vi "Updater.vi"() -> ()   [LabVIEW 2011]
uses:
  Summitek EXT/Miscellaneous/OGAB Version.ctl
  server/database/History/History Record.ctl
  server/database/Fields/Field Record.ctl
  server/database/Fields/Field DataTypes.ctl
  server/database/Fields/Field NextItem.ctl
  server/database/Stations/Instruments/Instrument Record Fields.ctl
  Summitek EXT/OpenG EXT/file/file.llb/File Exists - Scalar__ogtk.vi
  ITK EXT/http/config.llb/HTTP SRM.vi
panel:
  in  "spartan install path":path=path "C:/Development/Spartan"
  out "Database Operation":string
  out "Status":string
  out "Spartan Install Path":path
  out "ver":string
  in  "Version":T1 {"Build Date/Time" format="%<%X\n%x>T"}
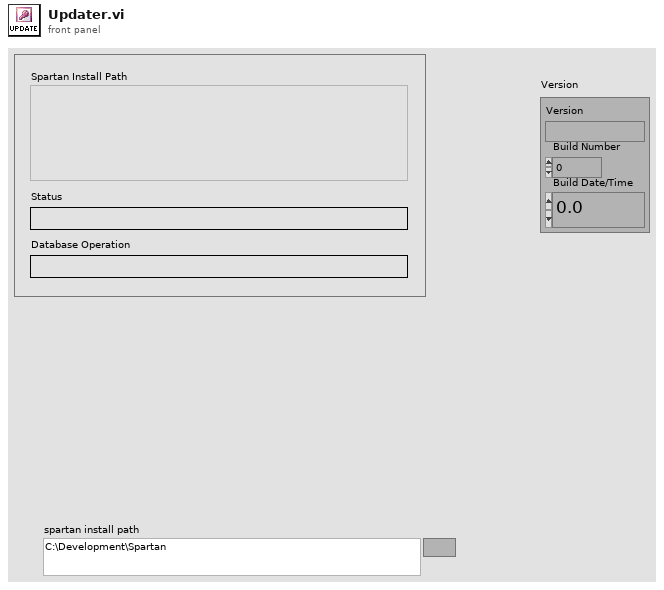
[diagram p1: front panel]
types:
  T1 = typedef "OGAB Version.ctl" = cluster{"Version":string, "Build Number":u32, "Build Date/Time":dbl}
  T2 = typedef "History Record.ctl" = cluster{"ixHistory":i32, "sVersion":string, "tUpdate":timestamp}
  T3 = typedef "Connection Refnum.ctl" = cluster{"Environment Handle":i32, "Connection Handle":i32}
  T4 = typedef "Field Record.ctl" = cluster{"ixField":i32, "iSequenceOrder":i32, "sxFieldId":string, "sxSequenceId":string, "sDisplayName":string, "sValue":string, "sUnits":string, "nDataType":T5, "nNextItem":T6, "fSystem":bool, "fSystemValue":bool, "fRequired":bool, "fSetAtTest":bool, "fTestField":bool, "fDeleted":bool, "fIndexed":bool, "fFreeList":bool}
  T5 = typedef "Field DataTypes.ctl" = enum32{"text", "numeric", "list", "timestamp", "boolean"}
  T6 = typedef "Field NextItem.ctl" = enum32{"Reset", "Retain", "Auto-Increment"}
  T7 = typedef "Instrument Record Fields.ctl" = enum32{"sxInstrumentId", "sDriverId", "sDriverType", "sSerialNumber", "tLastCalibration", "tCalibrationDue", "sConfiguration", "ixInstrument"}
  T8 = cluster{"Environment Handle":i32, "Connection Handle":i32}
  T9 = typedef "Instrument Record.ctl" = cluster{"ixInstrument":i32, "sxInstrumentId":string, "sDriverId":string, "sDriverType":string, "sSerialNumber":string, "tLastCalibration":timestamp, "tCalibrationDue":timestamp, "sConfiguration":string}
  T10 = cluster{"IndexName":string, "sxFieldId":string}[]
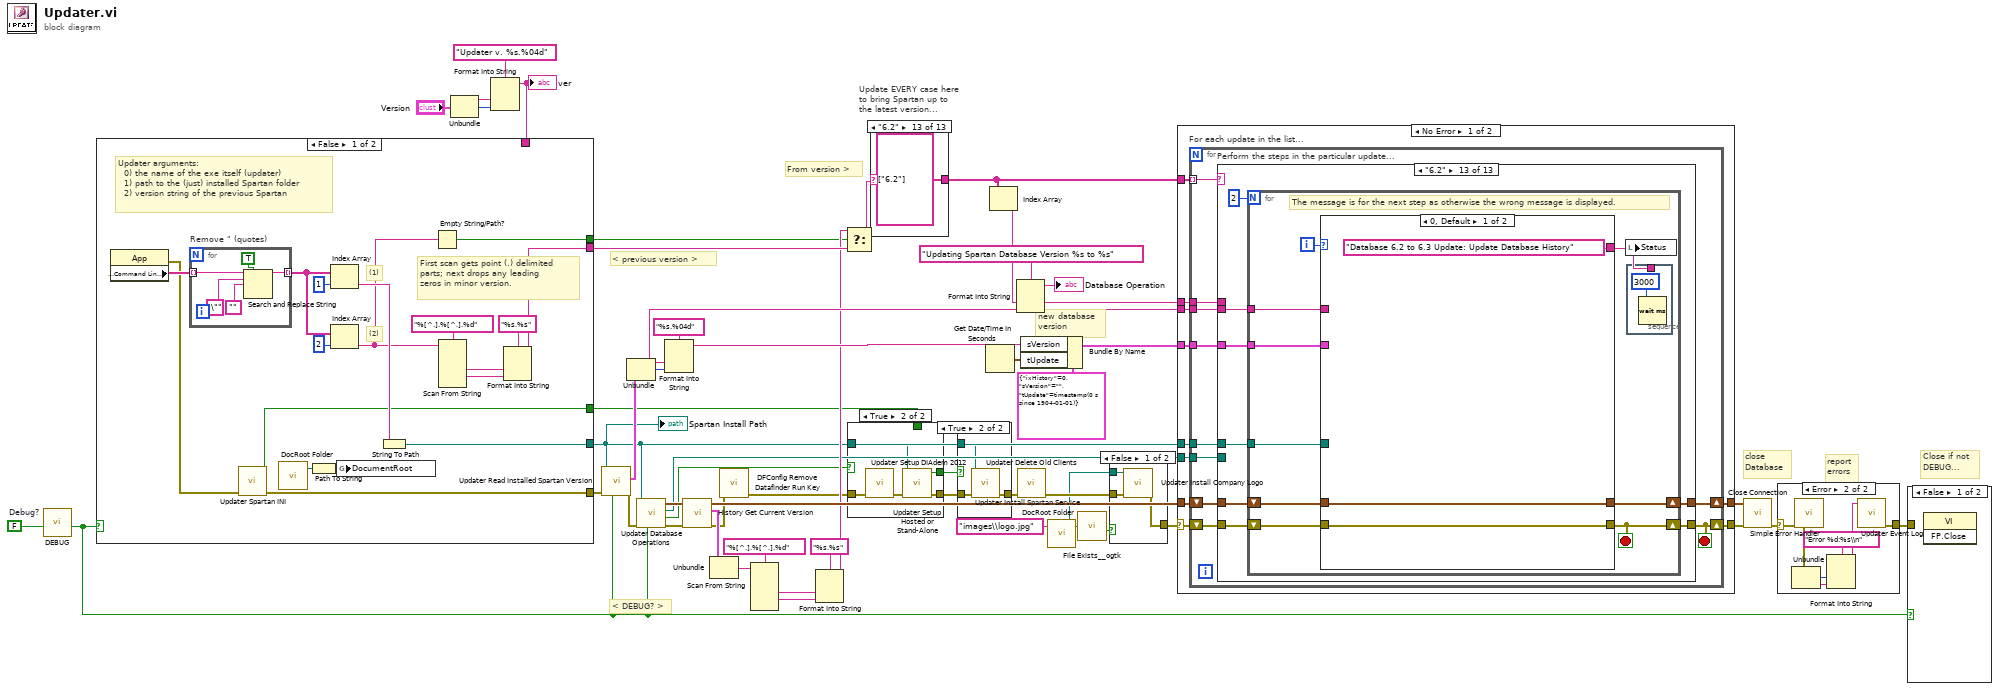
[diagram p0: block diagram]
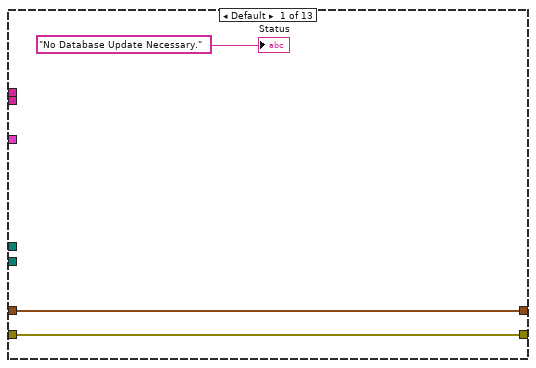
[diagram p2: hidden frame]
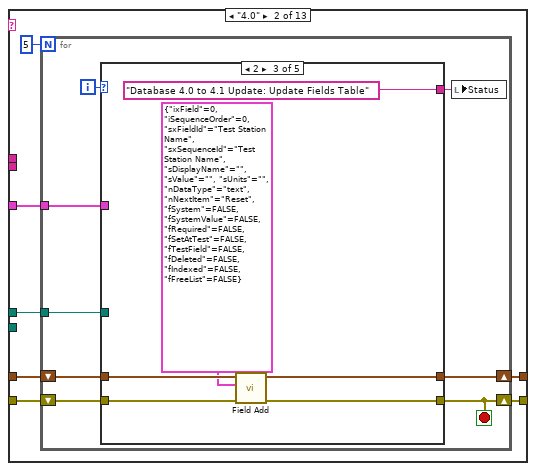
[diagram p3: hidden frame]
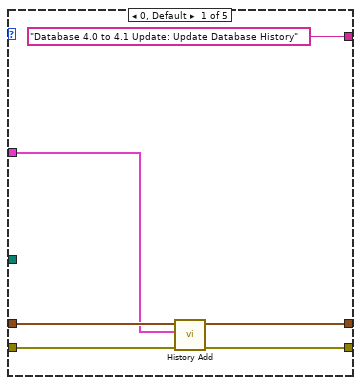
[diagram p4: hidden frame]
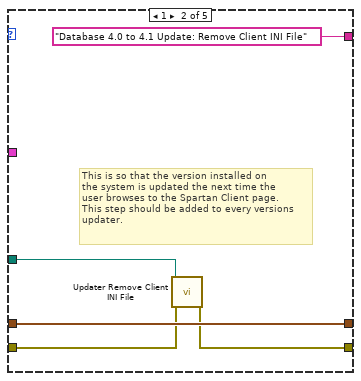
[diagram p5: hidden frame]
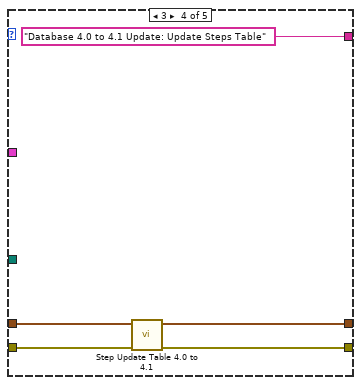
[diagram p6: hidden frame]
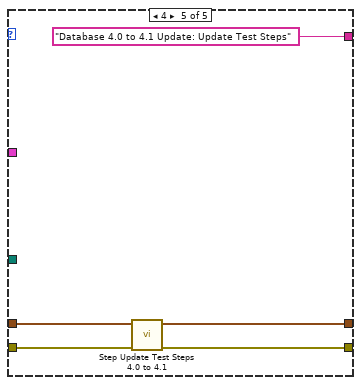
[diagram p7: hidden frame]
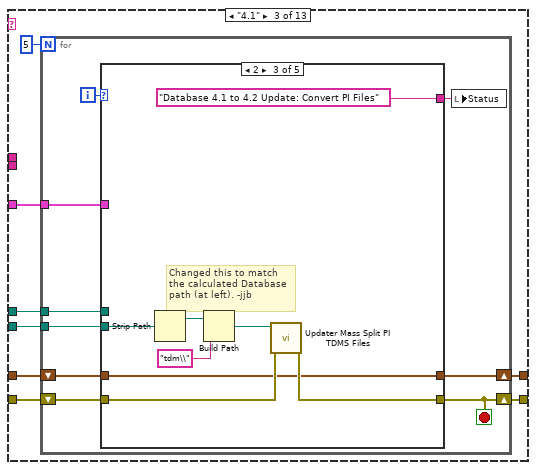
[diagram p8: hidden frame]
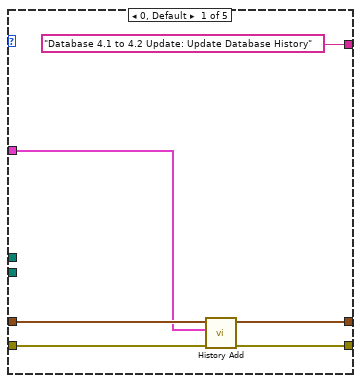
[diagram p9: hidden frame]
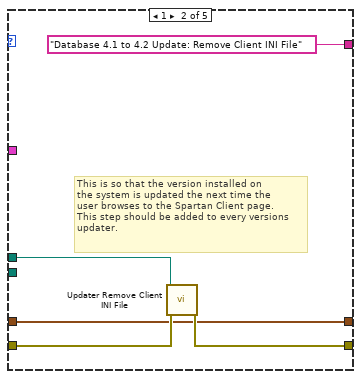
[diagram p10: hidden frame]
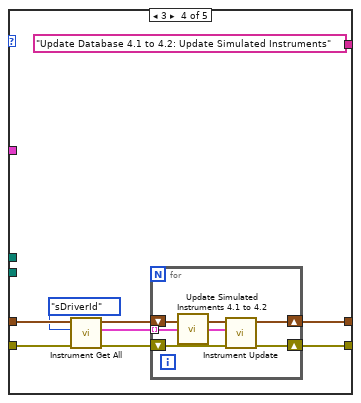
[diagram p11: hidden frame]
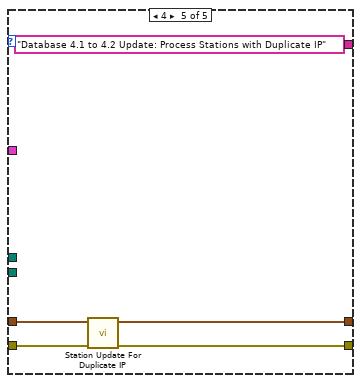
[diagram p12: hidden frame]
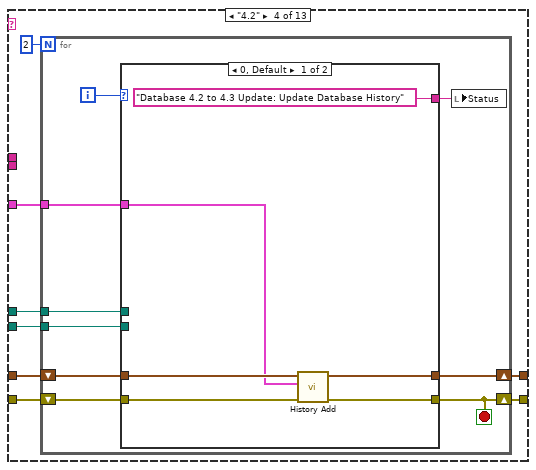
[diagram p13: hidden frame]
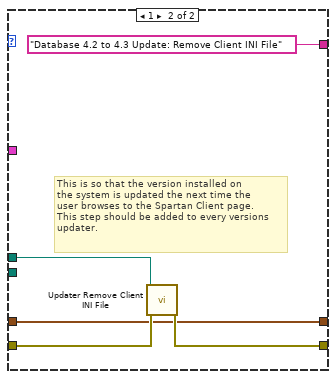
[diagram p14: hidden frame]
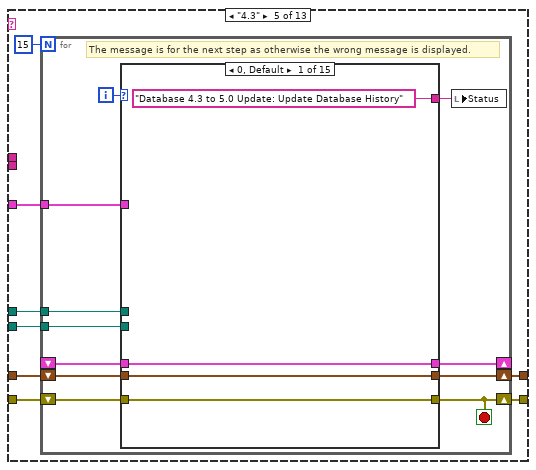
[diagram p15: hidden frame]
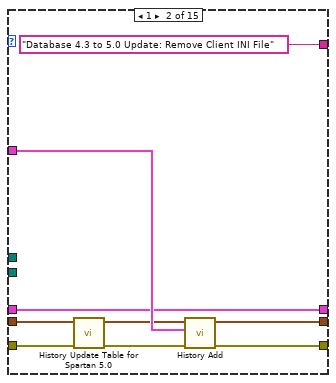
[diagram p16: hidden frame]
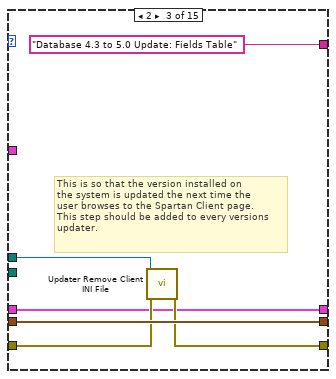
[diagram p17: hidden frame]
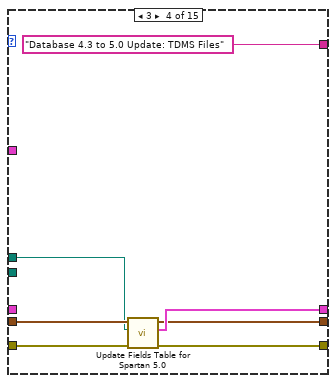
[diagram p18: hidden frame]
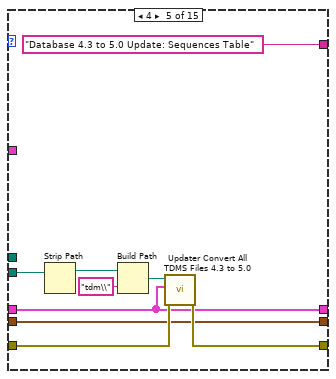
[diagram p19: hidden frame]
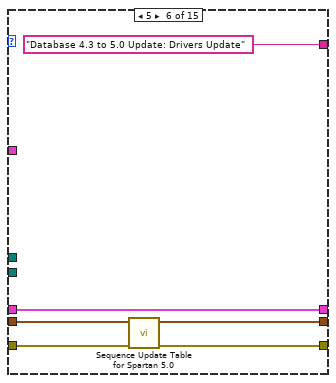
[diagram p20: hidden frame]
diagram:
  w47 = FALSE  # Debug?
  # "new database\nversion"
  # "From version >"
  # "close\nDatabase"
  # "report\nerrors"
  # "Close if not\nDEBUG..."
  # "< DEBUG? >"
  # "< previous version >"
  n1 = call "DEBUG.vi"("Dev DEBUG? (f)"=w47) -> ("DEBUG?"=w19:bool)  [unwired: 1 in, 5 out]
  n2 = Unbundle("Version") -> ("Version"=w50:string, "Build Number"=w51:u32)  [unwired: 1 out]
  n3 = Format Into String(format string="Updater v. %s.%04d", w50, w51) -> (resulting string=w45:string)  [unwired: 2 in, 1 out]
  "ver" <- w45
  n4 = case shown="False" w19 {
    tunnel: [w61 "spartan install path"] -> w9
    tunnel: [w63 "5.2"] -> w48
    tunnel: [w59 errorcluster {"status"=FALSE, "code"=0, "source"=""} ("error out")] -> w23
    tunnel: w45 -> [_ _]
    tunnel: [w56 TRUE] -> w15
    tunnel: [w55 _] -> w8
    frame False {
      # "First scan gets point (.) delimited\nparts; next drops any leading\nzeros in minor version."
      # "(2)"
      # "(1)"
      # "Updater arguments:\n  0) the name of the exe itself (updater)\n  1) path to the (just) installed Spartan folder\n  2) version string of the previous Spartan"
      n5 = property class="App"() -> (error out=w60:errorcluster, "Application:Command Line Arguments"=w70:string[])  [unwired: 2 in, 1 out]
      n6 = for "Remove \" (quotes)" {
        tunnel: w70 -> [w73] mode=indexing
        tunnel: [w72] -> w67 mode=indexing
        n7 = Search and Replace String(replace all?=TRUE, input string=w73, search string="\"", replace string="") -> (result string=w72:string)  [unwired: 1 in, 6 out]
      }
      n8 = call "Updater Spartan INI.vi"("error in (no error)"=w60) -> ("error out"=w59:errorcluster, "Run as Service?"=w55:bool)  [unwired: 9 in]
      n9 = call "DocRoot Folder.vi"() -> ("DocumentRoot Folder"=w54:path)  [unwired: 3 in]
      n10 = Path To String(path=w54) -> (string=w53:string)
      n11 = Index Array(array=w67, index=1) -> (element=w62:string)
      n12 = Index Array(array=w67, index=2) -> (element=w57:string)
      n13 = global write "HTTP SRM.vi" "DocumentRoot"(w53) -> ()
      n14 = String To Path(string=w62) -> (path=w61:path)
      n15 = Empty String/Path?(string/path=w57) -> (empty?=w56:bool)
      n16 = Scan From String(format string="%[^.].%[^.].%d", input string=w57) -> (output 1=w64:string, output 2=w58:string)  [unwired: 2 in, 7 out]
      n17 = Format Into String(format string="%s.%s", w64, w58) -> (resulting string=w63:string)  [unwired: 2 in, 1 out]
    }
    frame True {
      # "<--- DEBUGGING --->"
    }
  }
  "Spartan Install Path" <- w9
  n18 = call "Updater Read Installed Spartan Version.vi"("DEBUG? (f)"=w19, "error in (no error)"=w23, "Spartan Install Folder (empty)"=w9) -> ("error out"=w22:errorcluster, "Version"=w41:T1)  [unwired: 3 in, 4 out]
  n19 = Unbundle(w41) -> ("Version"=w33:string, "Build Number"=w43:u32)  [unwired: 1 out]
  n20 = call "Updater Database Operations.vi"("Debug (f)?"=w19, "error in (no error)"=w22, "Spartan Install Path (empty)"=w9) -> ("error out"=w21:errorcluster, "New Spartan"=w13:bool, "Spartan Database Path"=w14:path, "Connection Refnum"=w20:T3)  [unwired: 5 in]
  n21 = Format Into String(format string="%s.%04d", w33, w43) -> (resulting string=w37:string)  [unwired: 2 in, 1 out]
  n22 = call "History Get Current Version.vi"("error in (no error)"=w21, "Connection Refnum"=w20) -> ("error out"=w16:errorcluster, "Current Version Record"=w31:T2, "Connection Refnum"=w32:T3)  [unwired: 7 in]
  n23 = Unbundle(w31) -> ("sVersion"=w26:string)  [unwired: 2 out]
  n24 = call "DFConfig Remove Datafinder Run Key.vi"("error in (no error)"=w16) -> ("error out"=w7:errorcluster)  [unwired: 10 out]
  n25 = Scan From String(format string="%[^.].%[^.].%d", input string=w26) -> (output 1=w28:string, output 2=w27:string)  [unwired: 2 in, 7 out]
  n26 = Format Into String(format string="%s.%s", w28, w27) -> (resulting string=w25:string)  [unwired: 2 in, 1 out]
  n27 = Select(t=w25, s=w15, f=w48) -> (s? t:f=w24:string)
  n28 = case shown="True" w13 {
    tunnel: w7 -> [w81 w83]
    tunnel: w9 -> [_ w86]
    tunnel: [w81 w85] -> w11
    tunnel: [w80 w84] -> w12
    tunnel: w8 -> [w80 _]
    frame False {
    }
    frame True {
      n29 = call "Updater Setup DIAdem 2012.vi"("error in (no error)"=w83) -> ("error out"=w82:errorcluster)  [unwired: 10 in]
      n30 = call "Updater Setup Hosted or Stand-Alone.vi"("error in (no error)"=w82, "Spartan Install Path (empty)"=w86) -> ("error out"=w85:errorcluster, "Hosted?"=w84:bool)  [unwired: 8 in]
    }
  }
  n31 = case "Update EVERY case here\nto bring Spartan up to\nthe latest version..." shown="\"6.2\"" w24 {
    tunnel: [string[] ["New Installation"] string[] ["4.0", "4.1", "4.2", "4.3", "5.0", "5.1", "5.2", "5.3", "5.4", "6.0", "6.1", "6.2"] string[] ["4.1", "4.2", "4.3", "5.0", "5.1", "5.2", "5.3", "5.4", "6.0", "6.1", "6.2"] string[] ["4.2", "4.3", "5.0", "5.1", "5.2", "5.3", "5.4", "6.0", "6.1", "6.2"] string[] ["4.3", "5.0", "5.1", "5.2", "5.3", "5.4", "6.0", "6.1", "6.2"] string[] ["5.0", "5.1", "5.2", "5.3", "5.4", "6.0", "6.1", "6.2"] string[] ["5.1", "5.2", "5.3", "5.4", "6.0", "6.1", "6.2"] string[] ["5.2", "5.3", "5.4", "6.0", "6.1", "6.2"] string[] ["5.3", "5.4", "6.0", "6.1", "6.2"] string[] ["5.4", "6.0", "6.1", "62."] string[] ["6.0", "6.1", "6.2"] string[] ["6.1", "6.2"] string[] ["6.2"]] -> w2
    frame Default {
    }
    frame "4.0" {
    }
    frame "4.1" {
    }
    frame "4.2" {
    }
    frame "4.3" {
    }
    frame "5.0" {
    }
    frame "5.1" {
    }
    frame "5.2" {
    }
    frame "5.3" {
    }
    frame "5.4" {
    }
    frame "6.0" {
    }
    frame "6.1" {
    }
    frame "6.2" {
    }
  }
  n32 = case shown="True" w12 {
    tunnel: w11 -> [w100 w102]
    tunnel: [w100 w103] -> w10
    tunnel: w9 -> [_ w101]
    frame False {
    }
    frame True {
      n33 = call "Updater Install Spartan Service.vi"("error in (no error)"=w102, "Spartan Install Path"=w101) -> ("error out"=w103:errorcluster)  [unwired: 9 in]
    }
  }
  n34 = Get Date/Time In Seconds() -> (seconds since 1Jan1904=w40:timestamp)
  n35 = Index Array(array=w2) -> (element=w18:string)  [unwired: 1 in]
  n36 = Format Into String(format string="Updating Spartan Database Version %s to %s", w18, w33) -> (resulting string=→"Database Operation":string)  [unwired: 2 in, 1 out]
  n37 = call "Updater Delete Old Clients.vi"("error in (no error)"=w10) -> ("error out"=w6:errorcluster)  [unwired: 10 in]
  n38 = Bundle By Name(cluster=T2 {"ixHistory"=0, "sVersion"="", "tUpdate"=timestamp(0 s since 1904-01-01)} ("Auto_Number Record"), "sVersion"=w37, "tUpdate"=w40) -> (w38:T2)
  n39 = call "DocRoot Folder.vi"("Relative Path (\"\" - Folder)"="images\\logo.jpg" ("Relative Path (\"\" - Folder)")) -> ("DocumentRoot Folder"=w3:path)  [unwired: 2 in]
  n40 = call-poly "File Exists__ogtk.vi"("file path"=w3) -> ("exists"=w4:bool)  [unwired: 6 in, 1 out]
  n41 = case shown="False" w4 {
    tunnel: w6 -> [w106 w107]
    tunnel: [w105 w107] -> w1
    tunnel: w3 -> [w104 _]
    frame False {
      n42 = call "Updater Install Company Logo.vi"("error in (no error)"=w106, "Path to File"=w104) -> ("error out"=w105:errorcluster)  [unwired: 9 in]
    }
    frame True {
    }
  }
  n43 = case shown="No Error" w1 {
    selector: w1 -> [w108 w655]
    tunnel: w38 -> [w117 _]
    tunnel: [w116 w655] -> w36
    tunnel: [w115 w656] -> w35
    tunnel: w33 -> [w114 _]
    tunnel: w32 -> [w113 w656]
    tunnel: w18 -> [w112 _]
    tunnel: w14 -> [w111 _]
    tunnel: w9 -> [w110 _]
    tunnel: w2 -> [w109 _]
    frame No Error {
      n44 = for "For each update in the list..." {
        tunnel: w109 -> [w127] mode=indexing
        tunnel: w117 -> [w126]
        shift-right: [w123] -> w115
        shift-left: w113 -> [w125]
        shift-right: [w118] -> w116
        shift-left: w108 -> [w124]
        tunnel: w111 -> [w122]
        tunnel: w110 -> [w121]
        tunnel: w112 -> [w120]
        tunnel: w114 -> [w119]
        stop <- w118 stop-if-true
        n45 = case "Perform the steps in the particular update..." shown="\"6.2\"" w127 {
          tunnel: w124 -> [w129 w133 w178 w234 w262 w368 w416 w450 w490 w537 w582 w608 w634]
          tunnel: w125 -> [w128 w134 w177 w233 w261 w367 w415 w449 w489 w536 w581 w607 w633]
          tunnel: [w129 w135 w176 w232 w260 w366 w414 w448 w488 w535 w580 w606 w632] -> w118
          tunnel: w126 -> [_ w136 w179 w235 w263 w369 w417 w451 w491 w538 w583 w609 w635]
          tunnel: [w128 w132 w175 w231 w259 w365 w413 w447 w487 w534 w579 w605 w631] -> w123
          tunnel: w122 -> [_ _ w174 w230 w258 w364 _ _ _ _ _ _ _]
          tunnel: w121 -> [_ w131 w173 w229 w257 w363 _ w446 w486 w533 w578 w604 w630]
          tunnel: w120 -> [_ _ _ _ _ w362 _ _ _ _ _ _ _]
          tunnel: w119 -> [_ _ _ _ _ w361 w412 w445 w485 w532 w577 w603 w629]
          frame Default {
            "Status" <- "No Database Update Necessary." ("Status")
          }
          frame "4.0" {
            n46 = for {
              N: 5 -> [_]
              tunnel: w136 -> [w144]
              shift-right: [w138] -> w135
              shift-left: w133 -> [w141]
              shift-right: [w140] -> w132
              shift-left: w134 -> [w142]
              tunnel: w131 -> [w139]
              i -> [w145]
              stop <- w138 stop-if-true
              n47 = case shown="2" w145 {
                tunnel: w142 -> [w150 w155 w162 w165 w171]
                tunnel: w141 -> [w149 w154 w161 w166 w172]
                tunnel: [w151 w153 w160 w167 w169] -> w138
                tunnel: w144 -> [w146 _ _ _ _]
                tunnel: ["Database 4.0 to 4.1 Update: Update Database History" "Database 4.0 to 4.1 Update: Remove Client INI File" "Database 4.0 to 4.1 Update: Update Fields Table" "Database 4.0 to 4.1 Update: Update Steps Table" "Database 4.0 to 4.1 Update: Update Test Steps"] -> w143
                tunnel: [w147 w155 w157 w163 w168] -> w140
                tunnel: w139 -> [_ w152 _ _ _]
                frame 0, Default {
                  n48 = call "History Add.vi"("error in (no error)"=w149, "History Record"=w146, "Connection Refnum"=w150) -> ("error out"=w151:errorcluster, "Connection Refnum"=w147:T3)  [unwired: 7 out]
                }
                frame 1 {
                  # "This is so that the version installed on\nthe system is updated the next time the\nuser browses to the Spartan Client page.\nThis step should be added to every versions\nupdater."
                  n49 = call "Updater Remove Client INI File.vi"("error in (no error)"=w154, "Spartan Install Path"=w152) -> ("error out"=w153:errorcluster)  [unwired: 9 out]
                }
                frame 2 {
                  n50 = call "Field Add.vi"("error in (no error)"=w161, "Field Record"=T4 {"ixField"=0, "iSequenceOrder"=0, "sxFieldId"="Test Station Name", "sxSequenceId"="Test Station Name", "sDisplayName"="", "sValue"="", "sUnits"="", "nDataType"=enum."text", "nNextItem"=enum."Reset", "fSystem"=FALSE, "fSystemValue"=FALSE, "fRequired"=FALSE, "fSetAtTest"=FALSE, "fTestField"=FALSE, "fDeleted"=FALSE, "fIndexed"=FALSE, "fFreeList"=FALSE}, "Connection Refnum"=w162) -> ("error out"=w160:errorcluster, "Connection Refnum"=w157:T3)  [unwired: 1 in, 6 out]
                }
                frame 3 {
                  n51 = call "Step Update Table 4.0 to 4.1.vi"("error in (no error)"=w166, "Connection Refnum"=w165) -> ("error out"=w167:errorcluster, "Connection Refnum Out"=w163:T8)  [unwired: 8 out]
                }
                frame 4 {
                  n52 = call "Step Update Test Steps 4.0 to 4.1.vi"("error in (no error)"=w172, "Connection Refnum"=w171) -> ("error out"=w169:errorcluster, "Connection Refnum Out"=w168:T8)  [unwired: 8 out]
                }
              }
              n53 = local write "Status"(w143) -> ()
            }
          }
          frame "4.1" {
            n54 = for {
              N: 5 -> [_]
              tunnel: w179 -> [w188]
              shift-right: [w184] -> w175
              shift-left: w177 -> [w185]
              shift-right: [w181] -> w176
              shift-left: w178 -> [w186]
              tunnel: w174 -> [w183]
              tunnel: w173 -> [w182]
              i -> [w189]
              stop <- w181 stop-if-true
              n55 = case shown="2" w189 {
                tunnel: w185 -> [w194 w197 w205 w215 w227]
                tunnel: w186 -> [w193 w199 w207 w216 w228]
                tunnel: [w195 w198 w206 w212 w226] -> w181
                tunnel: w188 -> [w191 _ _ _ _]
                tunnel: ["Database 4.1 to 4.2 Update: Update Database History" "Database 4.1 to 4.2 Update: Remove Client INI File" "Database 4.1 to 4.2 Update: Convert PI Files" "Update Database 4.1 to 4.2: Update Simulated Instruments" "Database 4.1 to 4.2 Update: Process Stations with Duplicate IP"] -> w187
                tunnel: [w190 w197 w205 w210 w225] -> w184
                tunnel: w183 -> [_ _ w202 _ _]
                tunnel: w182 -> [_ w196 _ _ _]
                frame 0, Default {
                  n56 = call "History Add.vi"("error in (no error)"=w193, "History Record"=w191, "Connection Refnum"=w194) -> ("error out"=w195:errorcluster, "Connection Refnum"=w190:T3)  [unwired: 7 out]
                }
                frame 1 {
                  # "This is so that the version installed on\nthe system is updated the next time the\nuser browses to the Spartan Client page.\nThis step should be added to every versions\nupdater."
                  n57 = call "Updater Remove Client INI File.vi"("error in (no error)"=w199, "Spartan Install Path"=w196) -> ("error out"=w198:errorcluster)  [unwired: 9 out]
                }
                frame 2 {
                  # "Changed this to match\nthe calculated Database\npath (at left). -jjb"
                  n58 = Strip Path(path=w202) -> (stripped path=w203:path)  [unwired: 1 out]
                  n59 = Build Path(base path=w203, name or relative path="tdm\\") -> (appended path=w201:path)
                  n60 = call "Updater Mass Split PI TDMS Files.vi"("error in (no error)"=w207, "Spartan TDM Path"=w201) -> ("error out"=w206:errorcluster)  [unwired: 9 out]
                }
                frame 3 {
                  n61 = call "Instrument Get All.vi"("error in (no error)"=w216, "Sort by (sxInstrumentId)"=Instrument_Record_Fields."sDriverId" ("Sort by (Instrument_ID)"), "Connection Refnum"=w215) -> ("error out"=w213:errorcluster, "Instruments"=w209:T9[], "Connection Refnum"=w211:T3)  [unwired: 1 in, 5 out]
                  n62 = for {
                    shift-right: [w222] -> w212
                    shift-left: w213 -> [w223]
                    tunnel: w209 -> [w219] mode=indexing
                    shift-right: [w220] -> w210
                    shift-left: w211 -> [w221]
                    n63 = call "Update Simulated Instruments 4.1 to 4.2.vi"("Instrument Information"=w219) -> ("updated Instrument"=w218:T9)  [unwired: 2 in, 6 out]
                    n64 = call "Instrument Update.vi"("error in (no error)"=w223, "Instrument Record"=w218, "Connection Refnum"=w221) -> ("error out"=w222:errorcluster, "Connection Refnum"=w220:T3)  [unwired: 7 out]
                  }
                }
                frame 4 {
                  n65 = call "Station Update For Duplicate IP.vi"("error in (no error)"=w228, "Connection Refnum"=w227) -> ("error out"=w226:errorcluster, "Connection Refnum"=w225:T3)  [unwired: 8 out]
                }
              }
              n66 = local write "Status"(w187) -> ()
            }
          }
          frame "4.2" {
            n67 = for {
              N: 2 -> [_]
              tunnel: w235 -> [w244]
              shift-right: [w240] -> w231
              shift-left: w233 -> [w241]
              shift-right: [w237] -> w232
              shift-left: w234 -> [w242]
              tunnel: w230 -> [w239]
              tunnel: w229 -> [w238]
              i -> [w245]
              stop <- w237 stop-if-true
              n68 = case shown="0, Default" w245 {
                tunnel: w241 -> [w250 w253]
                tunnel: w242 -> [w249 w256]
                tunnel: [w251 w255] -> w237
                tunnel: w244 -> [w247 _]
                tunnel: ["Database 4.2 to 4.3 Update: Update Database History" "Database 4.2 to 4.3 Update: Remove Client INI File"] -> w243
                tunnel: [w246 w253] -> w240
                tunnel: w239 -> [_ _]
                tunnel: w238 -> [_ w252]
                frame 0, Default {
                  n69 = call "History Add.vi"("error in (no error)"=w249, "History Record"=w247, "Connection Refnum"=w250) -> ("error out"=w251:errorcluster, "Connection Refnum"=w246:T3)  [unwired: 7 out]
                }
                frame 1 {
                  # "This is so that the version installed on\nthe system is updated the next time the\nuser browses to the Spartan Client page.\nThis step should be added to every versions\nupdater."
                  n70 = call "Updater Remove Client INI File.vi"("error in (no error)"=w256, "Spartan Install Path"=w252) -> ("error out"=w255:errorcluster)  [unwired: 9 out]
                }
              }
              n71 = local write "Status"(w243) -> ()
            }
          }
          frame "4.3" {
            n72 = for {
              N: 15 -> [_]
              tunnel: w263 -> [w274]
              shift-right: [w270] -> w259
              shift-left: w261 -> [w271]
              shift-right: [w265] -> w260
              shift-left: w262 -> [w272]
              tunnel: w258 -> [w269]
              tunnel: w257 -> [w268]
              shift-right: [w267] -> _
              shift-left: _ -> [w266]
              i -> [w275]
              stop <- w265 stop-if-true
              # "The message is for the next step as otherwise the wrong message is displayed."
              n73 = case shown="0, Default" w275 {
                tunnel: w271 -> [w279 w283 w293 w297 w304 w311 w318 w323 w328 w333 w338 w343 w348 w353 w360]
                tunnel: w272 -> [w278 w282 w292 w300 w310 w315 w321 w326 w331 w336 w341 w346 w351 w356 w357]
                tunnel: [w278 w286 w291 w299 w309 w314 w320 w325 w330 w335 w340 w345 w350 w355 w358] -> w265
                tunnel: w274 -> [_ w288 _ _ _ _ _ _ _ _ _ _ _ _ _]
                tunnel: ["Database 4.3 to 5.0 Update: Update Database History" "Database 4.3 to 5.0 Update: Remove Client INI File" "Database 4.3 to 5.0 Update: Fields Table" "Database 4.3 to 5.0 Update: TDMS Files" "Database 4.3 to 5.0 Update: Sequences Table" "Database 4.3 to 5.0 Update: Drivers Update" "Database 4.3 to 5.0 Update: Tests Table" "Database 4.3 to 5.0 Update: Associations Table" "Database 4.3 to 5.0 Update: Instruments Table" "Database 4.3 to 5.0 Update: Stations Table" "Database 4.3 to 5.0 Update: Auto Number Table" "Database 4.3 to 5.0 Update: Users Table" "Database 4.3 to 5.0 Update: Steps Table" "Database 4.3 to 5.0 Update: Templates Table" _] -> w273
                tunnel: [w279 w287 w293 w296 w304 w312 w319 w324 w329 w334 w339 w344 w349 w354 w359] -> w270
                tunnel: w269 -> [_ _ _ _ w306 _ _ _ _ _ _ _ _ _ _]
                tunnel: w268 -> [_ _ w290 w295 _ _ _ _ _ _ _ _ _ _ _]
                tunnel: [w276 w284 w289 w298 w303 w313 _ _ _ _ _ _ _ _ _] -> w267
                tunnel: w266 -> [w276 w284 w289 _ w303 w313 _ _ _ _ _ _ _ _ _]
                frame 0, Default {
                }
                frame 1 {
                  n74 = call "History Update Table for Spartan 5.0.vi"("error in (no error)"=w282, "Connection Refnum"=w283) -> ("error out"=w280:errorcluster, "Connection Refnum"=w281:T3)  [unwired: 8 out]
                  n75 = call "History Add.vi"("error in (no error)"=w280, "History Record"=w288, "Connection Refnum"=w281) -> ("error out"=w286:errorcluster, "Connection Refnum"=w287:T3)  [unwired: 7 out]
                }
                frame 2 {
                  # "This is so that the version installed on\nthe system is updated the next time the\nuser browses to the Spartan Client page.\nThis step should be added to every versions\nupdater."
                  n76 = call "Updater Remove Client INI File.vi"("error in (no error)"=w292, "Spartan Install Path"=w290) -> ("error out"=w291:errorcluster)  [unwired: 9 out]
                }
                frame 3 {
                  n77 = call "Update Fields Table for Spartan 5.0.vi"("error in (no error)"=w300, "spartan install dir"=w295, "Connection Refnum"=w297) -> ("error out"=w299:errorcluster, "Map IndexName to FieldId"=w298:T10, "dup Connection Refnum"=w296:T3)  [unwired: 6 out]
                }
                frame 4 {
                  n78 = Strip Path(path=w306) -> (stripped path=w307:path)  [unwired: 1 out]
                  n79 = Build Path(base path=w307, name or relative path="tdm\\") -> (appended path=w305:path)
                  n80 = call "Updater Convert All TDMS Files 4.3 to 5.0.vi"("error in (no error)"=w310, "Map IndexName to FieldId"=w303, "Folder Path"=w305) -> ("error out"=w309:errorcluster)  [unwired: 8 out]
                }
                frame 5 {
                  n81 = call "Sequence Update Table for Spartan 5.0.vi"("error in (no error)"=w315, "Connection Refnum"=w311) -> ("error out"=w314:errorcluster, "Connection Refnum"=w312:T3)  [unwired: 8 out]
                }
                frame 6 {
                  n82 = call "Driver Update Table for Spartan 5.0.vi"("error in (no error)"=w321, "Connection Refnum"=w318) -> ("error out"=w320:errorcluster, "dup Connection Refnum"=w319:T3)  [unwired: 8 out]
                }
                frame 7 {
                  n83 = call "Test Update Table for Spartan 5.0.vi"("error in (no error)"=w326, "Connection Refnum"=w323) -> ("error out"=w325:errorcluster, "Connection Refnum"=w324:T3)  [unwired: 8 out]
                }
                frame 8 {
                  n84 = call "Association Update Table for Spartan 5.0.vi"("error in (no error)"=w331, "Connection Refnum"=w328) -> ("error out"=w330:errorcluster, "Connection Refnum"=w329:T3)  [unwired: 8 out]
                }
                frame 9 {
                  n85 = call "Instrument Update Table for Spartan 5.0.vi"("error in (no error)"=w336, "Connection Refnum"=w333) -> ("error out"=w335:errorcluster, "Connection Refnum"=w334:T3)  [unwired: 8 out]
                }
                frame 10 {
                  n86 = call "Station Update Table for Spartan 5.0.vi"("error in (no error)"=w341, "Connection Refnum"=w338) -> ("error out"=w340:errorcluster, "Connection Refnum"=w339:T3)  [unwired: 8 out]
                }
                frame 11 {
                  n87 = call "Auto Number Update Table for Spartan 5.0.vi"("error in (no error)"=w346, "Connection Refnum"=w343) -> ("error out"=w345:errorcluster, "Connection Refnum"=w344:T3)  [unwired: 8 out]
                }
                frame 12 {
                  n88 = call "User Update Table for Spartan 5.0.vi"("error in (no error)"=w351, "Connection Refnum"=w348) -> ("error out"=w350:errorcluster, "Connection Refnum"=w349:T3)  [unwired: 8 out]
                }
                frame 13 {
                  n89 = call "Step Update Table 4.3 to 5.0.vi"("error in (no error)"=w356, "Connection Refnum"=w353) -> ("error out"=w355:errorcluster, "Connection Refnum"=w354:T3)  [unwired: 8 out]
                }
                frame 14 {
                  n90 = call "Update Templates Table for Spartan 5.0.vi"("error in (no error)"=w357, "Connection Refnum"=w360) -> ("error out"=w358:errorcluster, "Connection Refnum"=w359:T3)  [unwired: 8 out]
                }
              }
              n91 = local write "Status"(w273) -> ()
            }
          }
          frame "5.0" {
            n92 = for {
              N: 5 -> [_]
              tunnel: w369 -> [w380]
              shift-right: [w376] -> w365
              shift-left: w367 -> [w377]
              shift-right: [w371] -> w366
              shift-left: w368 -> [w378]
              tunnel: w364 -> [w375]
              tunnel: w363 -> [w374]
              tunnel: w362 -> [w373]
              tunnel: w361 -> [w372]
              i -> [w381]
              stop <- w371 stop-if-true
              # "The message is for the next step as otherwise the wrong message is displayed."
              n93 = case shown="2" w381 {
                tunnel: w377 -> [w384 w386 w392 w405 w409]
                tunnel: w378 -> [w383 w385 w401 w407 w411]
                tunnel: [w383 w388 w400 w406 w410] -> w371
                tunnel: w380 -> [_ w390 _ _ _]
                tunnel: ["Database 5.0 to 5.1 Update: Update Database History" "Database 5.0 to 5.1 Update: TDMS Files" "Database 5.0 to 5.1 Update: Fields" "Database 5.0 to 5.1 Update: Steps" _] -> w379
                tunnel: [w384 w389 w391 w404 w408] -> w376
                tunnel: w375 -> [_ _ w397 _ _]
                tunnel: w374 -> [_ _ _ w403 _]
                tunnel: w373 -> [_ _ w394 _ _]
                tunnel: w372 -> [_ _ w393 _ _]
                frame 0, Default {
                }
                frame 1 {
                  n94 = call "History Add.vi"("error in (no error)"=w385, "History Record"=w390, "Connection Refnum"=w386) -> ("error out"=w388:errorcluster, "Connection Refnum"=w389:T3)  [unwired: 7 out]
                }
                frame 2 {
                  n95 = Strip Path(path=w397) -> (stripped path=w398:path)  [unwired: 1 out]
                  n96 = Build Path(base path=w398, name or relative path="tdm\\") -> (appended path=w396:path)
                  n97 = call "Updater Convert All TDMS Files 5.0 to 5.1.vi"("Current Version"=w393, "Connection Refnum In"=w392, "Previous Version"=w394, "error in (no error)"=w401, "Folder Path"=w396) -> ("error out"=w400:errorcluster, "Connection Refnum Out"=w391:T3)  [unwired: 5 out]
                }
                frame 3 {
                  n98 = call "Update Fields Table for Spartan 5.1.vi"("error in (no error)"=w407, "Spartan Install Dir"=w403, "Connection Refnum"=w405) -> ("error out"=w406:errorcluster, "Connection Refnum"=w404:T3)  [unwired: 7 out]
                }
                frame 4 {
                  n99 = call "Step Update Table 5.0 to 5.1.vi"("error in (no error)"=w411, "Connection Refnum"=w409) -> ("error out"=w410:errorcluster, "Connection Refnum"=w408:T3)  [unwired: 1 in, 7 out]
                }
              }
              n100 = local write "Status"(w379) -> ()
            }
          }
          frame "5.1" {
            n101 = for {
              N: 4 -> [_]
              tunnel: w417 -> [w425]
              shift-right: [w421] -> w413
              shift-left: w415 -> [w422]
              shift-right: [w419] -> w414
              shift-left: w416 -> [w423]
              tunnel: w412 -> [w420]
              i -> [w426]
              stop <- w419 stop-if-true
              # "The message is for the next step as otherwise the wrong message is displayed."
              n102 = case shown="0, Default" w426 {
                tunnel: w422 -> [w429 w431 w438 w442]
                tunnel: w423 -> [w428 w430 w440 w444]
                tunnel: [w428 w433 w439 w443] -> w419
                tunnel: w425 -> [_ w435 _ _]
                tunnel: ["Database 5.1 to 5.2 Update: Update Database History" "Database 5.1 to 5.2 Update: Fields" "Database 5.1 to 5.2 Update: Step Associations" _] -> w424
                tunnel: [w429 w434 w437 w441] -> w421
                tunnel: w420 -> [_ _ _ _]
                frame 0, Default {
                }
                frame 1 {
                  n103 = call "History Add.vi"("error in (no error)"=w430, "History Record"=w435, "Connection Refnum"=w431) -> ("error out"=w433:errorcluster, "Connection Refnum"=w434:T3)  [unwired: 7 out]
                }
                frame 2 {
                  n104 = call "Update Fields Table for Spartan 5.2.vi"("error in (no error)"=w440, "Connection Refnum"=w438) -> ("error out"=w439:errorcluster, "Connection Refnum"=w437:T3)  [unwired: 8 in]
                }
                frame 3 {
                  n105 = call "Update Add Step Associations Table for Spartan 5.2.vi"("error in (no error)"=w444, "Connection Refnum"=w442) -> ("error out"=w443:errorcluster, "Connection Refnum"=w441:T3)  [unwired: 8 in]
                }
              }
              n106 = local write "Status"(w424) -> ()
            }
          }
          frame "5.2" {
            n107 = for {
              N: 5 -> [_]
              tunnel: w451 -> [w460]
              shift-right: [w457] -> w447
              shift-left: w449 -> [w458]
              shift-right: [w453] -> w448
              shift-left: w450 -> [w459]
              tunnel: w446 -> [w456]
              tunnel: w445 -> [w455]
              i -> [w461]
              stop <- w453 stop-if-true
              # "The message is for the next step as otherwise the wrong message is displayed."
              n108 = case shown="0, Default" w461 {
                tunnel: w458 -> [w465 w467 w476 w479 w482]
                tunnel: w459 -> [w464 w466 w475 w481 w484]
                tunnel: [w464 w469 w473 w480 w483] -> w453
                tunnel: w460 -> [_ w471 _ _ _]
                tunnel: ["Database 5.2 to 5.3 Update: Update Database History" "Uninstall CrypKey Software" "Update S Parameter Fields Units" "Setup DIAdem 2010" _] -> w454
                tunnel: [w465 w470 w476 w478 w482] -> w457
                tunnel: w456 -> [_ _ w474 _ _]
                tunnel: w455 -> [_ _ _ _ _]
                frame 0, Default {
                }
                frame 1 {
                  n109 = call "History Add.vi"("error in (no error)"=w466, "History Record"=w471, "Connection Refnum"=w467) -> ("error out"=w469:errorcluster, "Connection Refnum"=w470:T3)  [unwired: 7 out]
                }
                frame 2 {
                  n110 = call "Updater Uninstall CrypKey.vi"("error in (no error)"=w475, "Spartan Install Path"=w474) -> ("error out"=w473:errorcluster)  [unwired: 9 in]
                }
                frame 3 {
                  n111 = call "Update Fields Table for Spartan 5.3.vi"("error in (no error)"=w481, "Connection Refnum"=w479) -> ("error out"=w480:errorcluster, "Connection Refnum"=w478:T3)  [unwired: 8 in]
                }
                frame 4 {
                  n112 = call "Updater Setup DIAdem 2012.vi"("error in (no error)"=w484) -> ("error out"=w483:errorcluster)  [unwired: 10 in]
                }
              }
              n113 = local write "Status"(w454) -> ()
              n114 = stacked-sequence {
                tunnel: w454 -> [_]
                frame #0 {
                  n115 = Wait (ms)(milliseconds to wait=u32 3000) -> ()  [unwired: 1 out]
                }
              }
            }
          }
          frame "5.3" {
            n116 = for {
              N: 6 -> [_]
              tunnel: w491 -> [w500]
              shift-right: [w497] -> w487
              shift-left: w489 -> [w498]
              shift-right: [w493] -> w488
              shift-left: w490 -> [w499]
              tunnel: w486 -> [w496]
              tunnel: w485 -> [w495]
              i -> [w501]
              stop <- w493 stop-if-true
              # "The message is for the next step as otherwise the wrong message is displayed."
              n117 = case shown="5" w501 {
                tunnel: w498 -> [w505 w509 w513 w520 w524 w529]
                tunnel: w499 -> [w504 w510 w512 w522 w527 w531]
                tunnel: [w504 w507 w515 w521 w526 w530] -> w493
                tunnel: w500 -> [_ _ w517 _ _ _]
                tunnel: ["Upgrade for Windows 7/2008 compatibility" "Database 5.3 to 5.4 Update: Update Database History" "Update Instruments Table" "Update S Parameter Fields Units" "Remove Duplicate Fields" _] -> w494
                tunnel: [w505 w508 w516 w519 w525 w528] -> w497
                tunnel: w496 -> [_ w506 _ _ _ _]
                tunnel: w495 -> [_ _ _ _ _ _]
                frame 0, Default {
                }
                frame 1 {
                  n118 = call "Updater Perform Upgrade to Winows 7-2008.vi"("Spartan Install Path"=w506, "error in (no error)"=w510, "Connection Refnum"=w509) -> ("error out"=w507:errorcluster, "Connection Refnum Out"=w508:T3)  [unwired: 7 in]
                }
                frame 2 {
                  n119 = call "History Add.vi"("error in (no error)"=w512, "History Record"=w517, "Connection Refnum"=w513) -> ("error out"=w515:errorcluster, "Connection Refnum"=w516:T3)  [unwired: 7 out]
                }
                frame 3 {
                  n120 = call "Instrument Update Table for Spartan 5.4.vi"("error in (no error)"=w522, "Connection Refnum"=w520) -> ("error out"=w521:errorcluster, "Connection Refnum"=w519:T3)  [unwired: 8 in]
                }
                frame 4 {
                  # "We need to redo this because it didn't happen\nin the 5.3 updater due to a bug."
                  n121 = call "Update Fields Table for Spartan 5.3.vi"("error in (no error)"=w527, "Connection Refnum"=w524) -> ("error out"=w526:errorcluster, "Connection Refnum"=w525:T3)  [unwired: 8 in]
                }
                frame 5 {
                  n122 = call "Fields Remove Duplicates.vi"("error in (no error)"=w531, "Connection Refnum"=w529) -> ("error out"=w530:errorcluster, "Connection Refnum"=w528:T3)  [unwired: 8 in]
                }
              }
              n123 = local write "Status"(w494) -> ()
              n124 = stacked-sequence {
                tunnel: w494 -> [_]
                frame #0 {
                  n125 = Wait (ms)(milliseconds to wait=u32 3000) -> ()  [unwired: 1 out]
                }
              }
            }
          }
          frame "5.4" {
            n126 = for {
              N: 6 -> [_]
              tunnel: w538 -> [w547]
              shift-right: [w544] -> w534
              shift-left: w536 -> [w545]
              shift-right: [w540] -> w535
              shift-left: w537 -> [w546]
              tunnel: w533 -> [w543]
              tunnel: w532 -> [w542]
              i -> [w548]
              stop <- w540 stop-if-true
              # "The message is for the next step as otherwise the wrong message is displayed."
              n127 = case shown="0, Default" w548 {
                tunnel: w545 -> [w551 w554 w561 w566 w571 w574]
                tunnel: w546 -> [w550 w553 w560 w565 w570 w575]
                tunnel: [w550 w556 w562 w567 w572 w576] -> w540
                tunnel: w547 -> [_ w558 _ _ _ _]
                tunnel: ["Database 5.4 to 6.0 Update: Update Database History" "Update Sequences Table" "Update Drivers" "Update Instruments" "Removing old drivers" _] -> w541
                tunnel: [w551 w557 w563 w568 w573 w574] -> w544
                tunnel: w543 -> [_ _ _ _ _ _]
                tunnel: w542 -> [_ _ _ _ _ _]
                frame 0, Default {
                }
                frame 1 {
                  n128 = call "History Add.vi"("error in (no error)"=w553, "History Record"=w558, "Connection Refnum"=w554) -> ("error out"=w556:errorcluster, "Connection Refnum"=w557:T3)  [unwired: 7 out]
                }
                frame 2 {
                  n129 = call "Sequence Update Table for Spartan 6.0.vi"("error in (no error)"=w560, "Connection Refnum"=w561) -> ("error out"=w562:errorcluster, "Connection Refnum"=w563:T3)  [unwired: 8 in]
                }
                frame 3 {
                  n130 = call "Driver Update sxDriverId for Spartan 6.0.vi"("error in (no error)"=w565, "Connection Refnum"=w566) -> ("error out"=w567:errorcluster, "Connection Refnum"=w568:T3)  [unwired: 8 in]
                }
                frame 4 {
                  n131 = call "Instrument Update sDriverId for Spartan 6.0.vi"("error in (no error)"=w570, "Connection Refnum"=w571) -> ("error out"=w572:errorcluster, "Connection Refnum"=w573:T3)  [unwired: 8 in]
                }
                frame 5 {
                  n132 = call "Driver Remove Summitek Drivers for Spartan 6.0.vi"("error in (no error)"=w575) -> ("error out"=w576:errorcluster)  [unwired: 10 in]
                }
              }
              n133 = local write "Status"(w541) -> ()
              n134 = stacked-sequence {
                tunnel: w541 -> [_]
                frame #0 {
                  n135 = Wait (ms)(milliseconds to wait=u32 3000) -> ()  [unwired: 1 out]
                }
              }
            }
          }
          frame "6.0" {
            n136 = for {
              N: 2 -> [_]
              tunnel: w583 -> [w592]
              shift-right: [w589] -> w579
              shift-left: w581 -> [w590]
              shift-right: [w585] -> w580
              shift-left: w582 -> [w591]
              tunnel: w578 -> [w588]
              tunnel: w577 -> [w587]
              i -> [w593]
              stop <- w585 stop-if-true
              # "The message is for the next step as otherwise the wrong message is displayed."
              n137 = case shown="0, Default" w593 {
                tunnel: w590 -> [w596 w599]
                tunnel: w591 -> [w595 w598]
                tunnel: [w595 w600] -> w585
                tunnel: w592 -> [_ w602]
                tunnel: ["Database 6.0 to 6.1 Update: Update Database History" _] -> w586
                tunnel: [w596 w601] -> w589
                tunnel: w588 -> [_ _]
                tunnel: w587 -> [_ _]
                frame 0, Default {
                }
                frame 1 {
                  n138 = call "History Add.vi"("error in (no error)"=w598, "History Record"=w602, "Connection Refnum"=w599) -> ("error out"=w600:errorcluster, "Connection Refnum"=w601:T3)  [unwired: 7 out]
                }
              }
              n139 = local write "Status"(w586) -> ()
              n140 = stacked-sequence {
                tunnel: w586 -> [_]
                frame #0 {
                  n141 = Wait (ms)(milliseconds to wait=u32 3000) -> ()  [unwired: 1 out]
                }
              }
            }
          }
          frame "6.1" {
            n142 = for {
              N: 2 -> [_]
              tunnel: w609 -> [w618]
              shift-right: [w615] -> w605
              shift-left: w607 -> [w616]
              shift-right: [w611] -> w606
              shift-left: w608 -> [w617]
              tunnel: w604 -> [w614]
              tunnel: w603 -> [w613]
              i -> [w619]
              stop <- w611 stop-if-true
              # "The message is for the next step as otherwise the wrong message is displayed."
              n143 = case shown="0, Default" w619 {
                tunnel: w616 -> [w622 w625]
                tunnel: w617 -> [w621 w624]
                tunnel: [w621 w626] -> w611
                tunnel: w618 -> [_ w628]
                tunnel: ["Database 6.1 to 6.2 Update: Update Database History" _] -> w612
                tunnel: [w622 w627] -> w615
                tunnel: w614 -> [_ _]
                tunnel: w613 -> [_ _]
                frame 0, Default {
                }
                frame 1 {
                  n144 = call "History Add.vi"("error in (no error)"=w624, "History Record"=w628, "Connection Refnum"=w625) -> ("error out"=w626:errorcluster, "Connection Refnum"=w627:T3)  [unwired: 7 out]
                }
              }
              n145 = local write "Status"(w612) -> ()
              n146 = stacked-sequence {
                tunnel: w612 -> [_]
                frame #0 {
                  n147 = Wait (ms)(milliseconds to wait=u32 3000) -> ()  [unwired: 1 out]
                }
              }
            }
          }
          frame "6.2" {
            n148 = for {
              N: 2 -> [_]
              tunnel: w635 -> [w644]
              shift-right: [w641] -> w631
              shift-left: w633 -> [w642]
              shift-right: [w637] -> w632
              shift-left: w634 -> [w643]
              tunnel: w630 -> [w640]
              tunnel: w629 -> [w639]
              i -> [w645]
              stop <- w637 stop-if-true
              # "The message is for the next step as otherwise the wrong message is displayed."
              n149 = case shown="0, Default" w645 {
                tunnel: w642 -> [w648 w651]
                tunnel: w643 -> [w647 w650]
                tunnel: [w647 w652] -> w637
                tunnel: w644 -> [_ w654]
                tunnel: ["Database 6.2 to 6.3 Update: Update Database History" _] -> w638
                tunnel: [w648 w653] -> w641
                tunnel: w640 -> [_ _]
                tunnel: w639 -> [_ _]
                frame 0, Default {
                }
                frame 1 {
                  n150 = call "History Add.vi"("error in (no error)"=w650, "History Record"=w654, "Connection Refnum"=w651) -> ("error out"=w652:errorcluster, "Connection Refnum"=w653:T3)  [unwired: 7 out]
                }
              }
              n151 = local write "Status"(w638) -> ()
              n152 = stacked-sequence {
                tunnel: w638 -> [_]
                frame #0 {
                  n153 = Wait (ms)(milliseconds to wait=u32 3000) -> ()  [unwired: 1 out]
                }
              }
            }
          }
        }
      }
    }
    frame Error {
    }
  }
  n154 = call "Close Connection.vi"("error in (no error)"=w36, "Connection Refnum"=w35) -> ("error out"=w17:errorcluster)  [unwired: 5 out]
  n155 = case shown="Error" w17 {
    selector: w17 -> [w657 w662]
    tunnel: [w657 w663] -> w52
    frame No Error {
    }
    frame Error {
      n156 = Unbundle(w662) -> ("code"=w660:i32, "source"=w659:string)  [unwired: 1 out]
      n157 = call <vilib>:"Simple Error Handler.vi"("error in (no error)"=w662) -> ()  [unwired: 1 in, 8 out]
      n158 = Format Into String(format string="Error %d:%s\\n" ("pattern"), w660, w659) -> (resulting string=w658:string)  [unwired: 2 in, 1 out]
      n159 = call "Updater Event Log.vi"("Log Entry"=w658) -> ("error out"=w663:errorcluster)  [unwired: 1 in, 9 out]
    }
  }
  n160 = case shown="False" w19 {
    tunnel: w52 -> [_ _]
    frame False {
      n161 = invoke class="VI" method="FP.Close"() -> ()  [unwired: 3 in, 3 out]
    }
    frame True {
    }
  }
